vi "Thermal Chamber Controller_DQMH_Action Update Set Point-with.queue-setup.vi"(11 "test case ID":string) -> (0 "error in":errorcluster, 3 "Temperature Set Point":dbl)   [LabVIEW 2018]
doc: "The setup VI should be executed before the VI under test in the harness VI. In this VI you can prepare the environment and the inputs of the VI under test.\n\nSee the Help Document for more information. (<b>Help</b> > <b>IncQuery Labs</b> > <b>InstaCoverage</b> > <b>InstaCoverage Help...</b>)"
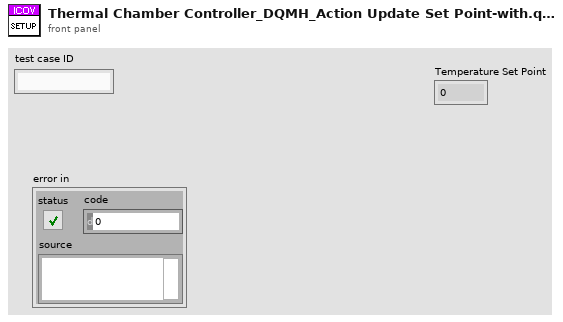
[diagram p1: front panel]
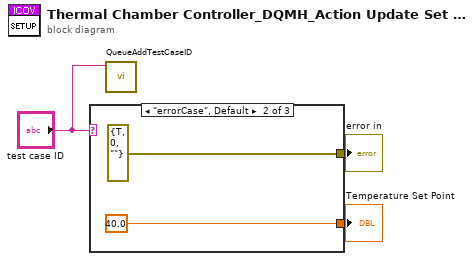
[diagram p0: block diagram]
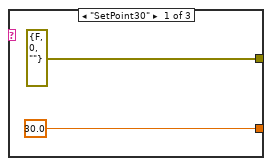
[diagram p2: hidden frame]
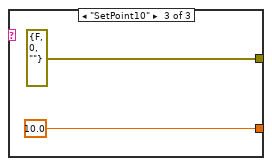
[diagram p3: hidden frame]
diagram:
  n1 = case shown="\"errorCase\", Default" "test case ID" {
    tunnel: [errorcluster {"status"=FALSE, "code"=0, "source"=""} ("error in (no error)") errorcluster {"status"=TRUE, "code"=0, "source"=""} ("error in (no error)") errorcluster {"status"=FALSE, "code"=0, "source"=""} ("error in (no error)")] -> w3
    tunnel: [30.0 ("Temperature Set Point") 40.0 ("Temperature Set Point") 10.0 ("Temperature Set Point")] -> w2
    frame "SetPoint30" {
    }
    frame "errorCase", Default {
    }
    frame "SetPoint10" {
    }
  }
  "error in" <- w3
  "Temperature Set Point" <- w2
  n2 = call "QueueAddTestCaseID.vi"("test case ID"="test case ID") -> ()  [unwired: 11 in]
